vi "Read Balance.vi"(8 "error in (no error)":errorcluster, 11 "AAccount in":refnum<class "AAccount.lvclass">) -> (0 "error out":errorcluster, 2 "Balance":dbl, 3 "AAccount out":refnum<class "AAccount.lvclass">)   [LabVIEW 2020, in "AAccount.lvclass"]
uses:
  AAccount.lvclass
  AAccount.lvclass/AAccount.ctl
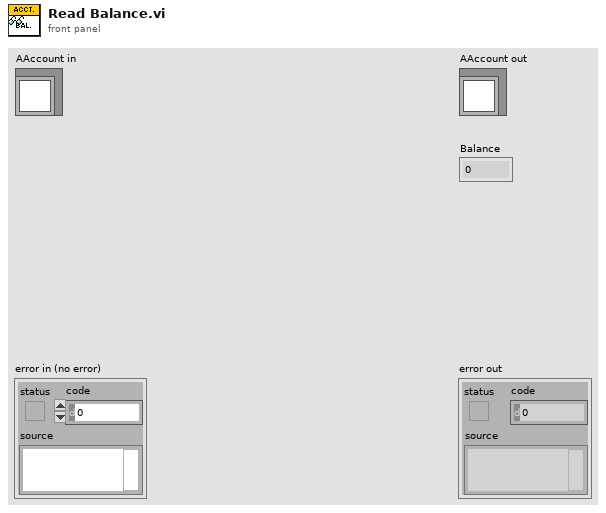
[diagram p1: front panel]
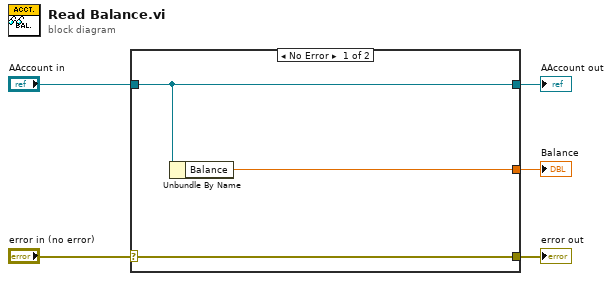
[diagram p0: block diagram]
diagram:
  n1 = case shown="No Error" "error in (no error)" {
    selector: "error in (no error)" -> [w8 w9]
    tunnel: [w8 w9] -> w4
    tunnel: [w7 w10] -> w2
    tunnel: "AAccount in" -> [w7 w10]
    tunnel: [w6 _] -> w1
    frame No Error {
      n2 = Unbundle By Name(w7) -> ("Balance"=w6:dbl)
    }
    frame Error {
    }
  }
  "error out" <- w4
  "AAccount out" <- w2
  "Balance" <- w1
